vi "Read Msg Attributes.vi"(11 "Base Actor in":refnum<class "Base Actor.lvclass">) -> (2 "Msg Attributes":refnum<data-value>)   [LabVIEW 2020, in "jettl.lvlib" / "Base jettl Actor.lvlib" / "Base Actor.lvlib" / "Base Actor.lvclass"]
uses:
  Base Actor.lvclass
  Base Actor.lvclass/Base Actor.ctl
  Msg/Msg.lvclass
  Relation.ctl
  jettl.lvlib
  Teller.ctl
  Msg Attributes.ctl
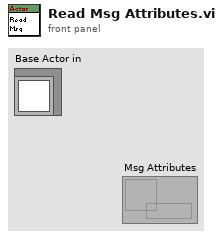
[diagram p1: front panel]
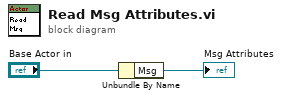
[diagram p0: block diagram]
diagram:
  n1 = Unbundle By Name("Base Actor in") -> ("Msg"=→"Msg Attributes":refnum<class "Msg.lvclass">)
